vi "空载速度.vi"(7 "枚举":enum16{"Read", "Write"}(ring), 11 "Status_Write":i16) -> (3 "Status_Read":sgl)   [LabVIEW 2020]
uses:
  Libraries/S7/S7.lvlib
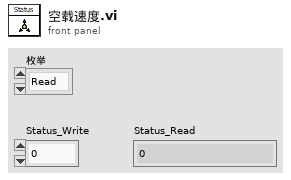
[diagram p1: front panel]
types:
  T1 = typedef "S7.lvlib/Read_Data (Reply Payload)--cluster.ctl" = cluster{"读取成功":bool, "数据":u32[], "Read_Data_error":errorcluster}
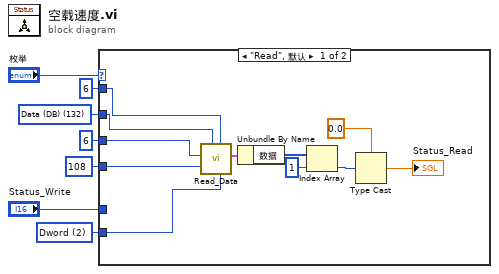
[diagram p0: block diagram]
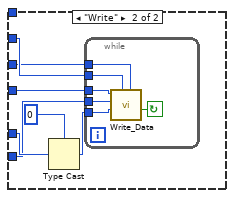
[diagram p2: hidden frame]
diagram:
  w3 = u16 2 items=["byte", "word", "Dword"] ("数据类型")
  w4 = u8 132 items=["I/O (P)"=128, "Input (I)"=129, "Output (Q)"=130, "Bit Memory (M)"=131, "Data (DB)"=132, "Instance Data (DI)"=133, "Local Data (L)"=134, "Predecessor Local Data (VL)"=135] ("寄存器类型")
  n1 = case shown="\"Read\", 默认" "枚举" {
    tunnel: u16 6 ("DB #") -> [w18 w20]
    tunnel: u32 108 ("起始地址") -> [w17 w19]
    tunnel: w4 -> [w16 w22]
    tunnel: u16 6 ("读取长度") -> [w15 _]
    tunnel: w3 -> [w14 w21]
    tunnel: "Status_Write" -> [_ w23]
    frame "Read", Default {
      n2 = call "Read_Data.vi"("数据类型"=w14, "读取长度"=w15, "寄存器类型"=w16, "起始地址"=w17, "DB #"=w18) -> ("Reply Payload"=w12:T1)  [unwired: 4 in, 2 out]
      n3 = Unbundle By Name(w12) -> ("数据"=w11:u32[])
      n4 = Index Array(array=w11, index=1 ("索引")) -> (element=w9:u32)
      n5 = Type Cast(type=0.0, x=w9) -> (*(type *) &x=→"Status_Read":dbl)
    }
    frame "Write" {
      n6 = Type Cast(type=u16 0, x=w23) -> (*(type *) &x=w24:u16)
      n7 = while {
        tunnel: w24 -> [w31]
        tunnel: w22 -> [w30]
        tunnel: w21 -> [w29]
        tunnel: w20 -> [w28]
        tunnel: w19 -> [w27]
        stop <- w26 continue-if-true
        n8 = call "Write_Data.vi"("DB #"=w28, "寄存器类型"=w30, "写入数据"=w31, "数据类型"=w29, "写入地址"=w27) -> ("timed out?"=w26:bool)  [unwired: 4 in, 2 out]
      }
    }
  }
